vi "_checkForUniqueName.vi"(7 "Replace?":bool, 8 "error in (no error)":errorcluster, 10 "Name":string, 11 "tBSONDocument in":refnum<class "tBSONDocument.lvclass">) -> (0 "error out":errorcluster, 2 "Replace Index":i32, 3 "tBSONDocument out":refnum<class "tBSONDocument.lvclass">)   [LabVIEW 2013, in "BSON.lvlib" / "tBSONDocument.lvclass"]
doc: "Checks to see if a given name is in this document. Returns an error if a replacement is not being attempted. If a replacement is being attempted it returns the index of the element to be replaced."
uses:
  tBSONDocument.lvclass
  tBSONDocument.lvclass/tBSONDocument.ctl
  status.ctl
  BSON.lvlib
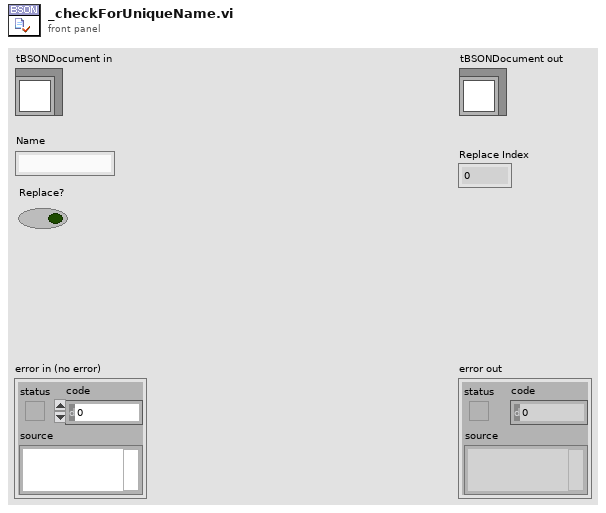
[diagram p1: front panel]
types:
  T1 = typedef "BSON.lvlib/status.ctl" = enum16{"Stream Corrupted or Ended Abruptly", "Incorrect Type In Stream", "ObjectID Invalid", "Method Not Implemented", "Invalid Name", "Invalid URI", "AutoReconnect", "Operation Failed", "Incorrectly Configured", "Cursor Not Found", "Timeout", "Invalid Type", "Empty Name", "Duplicate Name", "MD5Incorrect"}
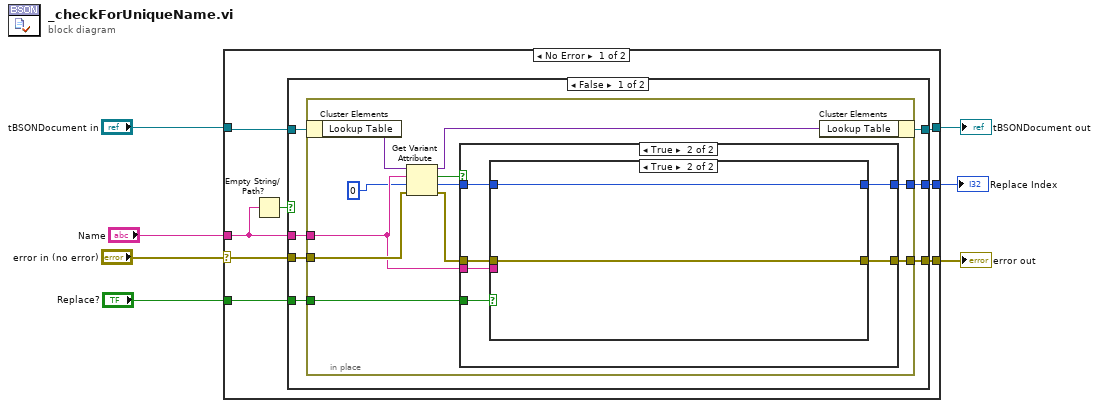
[diagram p0: block diagram]
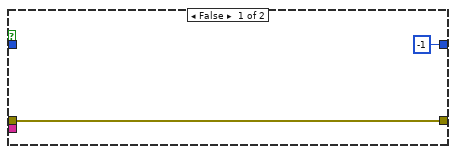
[diagram p2: hidden frame]
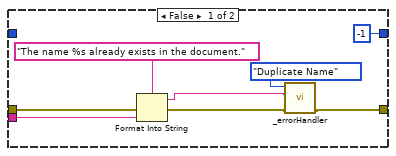
[diagram p3: hidden frame]
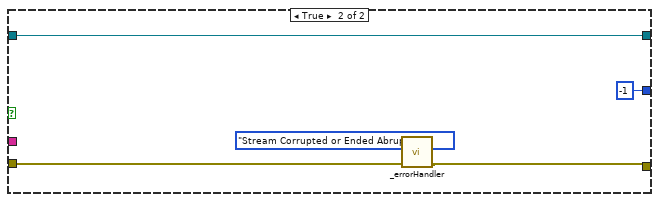
[diagram p4: hidden frame]
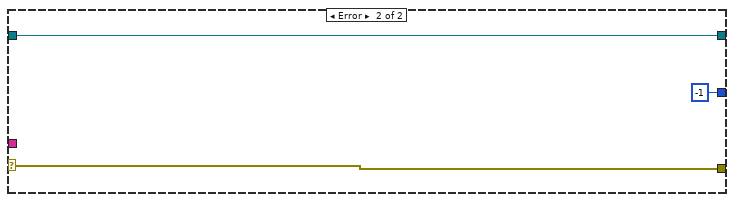
[diagram p5: hidden frame]
diagram:
  n1 = case shown="No Error" "error in (no error)" {
    selector: "error in (no error)" -> [w15 w59]
    tunnel: [w12 w59] -> w6
    tunnel: [w13 w58] -> w4
    tunnel: "tBSONDocument in" -> [w14 w58]
    tunnel: "Name" -> [w11 _]
    tunnel: "Replace?" -> [w9 _]
    tunnel: [w8 -1] -> w1
    frame No Error {
      n2 = Empty String/Path?(string/path=w11) -> (empty?=w10:bool)
      n3 = case shown="False" w10 {
        tunnel: w15 -> [w22 w55]
        tunnel: w14 -> [w21 w56]
        tunnel: [w20 w56] -> w13
        tunnel: [w19 w54] -> w12
        tunnel: w11 -> [w18 _]
        tunnel: w9 -> [w17 _]
        tunnel: [w16 -1] -> w8
        frame False {
          n4 = in-place {
            in-place-border: w18 -> [w28]
            in-place-border: w22 -> [w33]
            in-place-border: [w27] -> w19
            in-place-border: w17 -> [w26]
            in-place-border: [w23] -> w16
            n5 = in-place-cluster #1(w21) -> ("Lookup Table"=w30:variant)
            n6 = Get Variant Attribute(Variant=w30, name=w28, default value (empty Variant)=0, error in=w33) -> (duplicate Variant=w29:variant, found=w32:bool, value=w24:i32, error out=w31:errorcluster)
            n7 = case shown="True" w32 {
              tunnel: w31 -> [w35 w41]
              tunnel: w28 -> [_ w40]
              tunnel: [w35 w39] -> w27
              tunnel: w26 -> [_ w38]
              tunnel: w24 -> [_ w37]
              tunnel: [-1 w36] -> w23
              frame False {
              }
              frame True {
                n8 = case shown="True" w38 {
                  tunnel: w41 -> [w48 w50]
                  tunnel: w40 -> [w47 _]
                  tunnel: [w45 w50] -> w39
                  tunnel: w37 -> [_ w51]
                  tunnel: [-1 w51] -> w36
                  frame False {
                    n9 = Format Into String(format string="The name %s already exists in the document.", error in=w48, w47) -> (resulting string=w44:string, error out=w46:errorcluster)  [unwired: 1 in]
                    n10 = call "_errorHandler.vi"("error in (no error)"=w46, "Additional Text"=w44, "Error Type"=status."Duplicate Name") -> ("error out"=w45:errorcluster)  [unwired: 8 in]
                  }
                  frame True {
                  }
                }
              }
            }
            n11 = in-place-cluster #1("Lookup Table"=w29) -> (w20:refnum<class "tBSONDocument.lvclass">)
          }
        }
        frame True {
          n12 = call "_errorHandler.vi"("error in (no error)"=w55, "Error Type"=status."Stream Corrupted or Ended Abruptly") -> ("error out"=w54:errorcluster)  [unwired: 9 in]
        }
      }
    }
    frame Error {
    }
  }
  "error out" <- w6
  "tBSONDocument out" <- w4
  "Replace Index" <- w1
